vi "Simulation iRobot Sensors.vi"(8 "error in":errorcluster, 9 "Feedback Input":T1, 10 "Robot":T2, 11 "simulator":T16={"configuration"={"maxTime"=5.0, "enableVisualization"=TRUE, "Environment Definition"=path "simulation configuration.ini", "Record Location"=path "Simulation Record.xml", "autograde?"=TRUE, "interactive?"=FALSE, "Feedback Mode"=enum."debug navigation", "Robot State Charts"=[path "C:/Users/blueuser/Desktop/Robo Sim Berkley/cpsgrader-release-0.4/Simulators/EECS149lab/src/LabVIEW/statechart/Simulation Statechart.vi"], "statechart"=path "C:/Users/blueuser/Desktop/Robo Sim Berkley/cpsgrader-release-0.4/Simulators/EECS149lab/src/LabVIEW/statechart/Simulation Statechart.vi"}, "Statechart\ndisplay"=refnum, "first step?"=FALSE, "Robots Simulation Statecharts"=[], "Robots"=[]}) -> (0 "error out":errorcluster, 1 "Feedback Output":T1, 2 "sensors":T3={"net distance (mm)"=0, "net angle (deg)"=0, "accelerometer"={"x axis (g)"=0.0, "y axis (g)"=0.0, "z axis (g)"=0.0}, "iRobot Sensors"={"Bumps + Wheel Drops"={"Wheeldrop Caster"=FALSE, "Wheeldrop Left"=FALSE, "Wheeldrop Right"=FALSE, "Bump Left"=FALSE, "Bump Right"=FALSE}, "Wall"=FALSE, "Cliff Left"=FALSE, "Cliff Front Left"=FALSE, "Cliff Front Right"=FALSE, "Cliff Right"=FALSE, "Wall Signal"=0, "Cliff Left Signal"=0, "Cliff Front Left Signal"=0, "Cliff Front Right Signal"=0, "Cliff Right Signal"=0, "Buttons"={"Advance"=FALSE, "Play"=FALSE}, "Virtual Wall"=FALSE, "# Stream Packets"=0, "Requested Velocity (mm/s)"=0, "Requested Radius (mm)"=0, "Requested Right Wheel Velocity (mm/s)"=0, "Requested Left Wheel Velocity (mm/s)"=0, "Distance (mm)"=0, "Angle (deg)"=0, "Song Playing"=FALSE, "Song Number"=0, "Charging State"=enum."Not Charging", "Voltage (mV)"=0, "Current (mA)"=0, "Battery Temperature (deg C)"=0, "Battery Charge (mAh)"=0, "Battery Capacity (mAh)"=0, "Charging Sources"={"Internal Charger"=FALSE, "Home Base"=FALSE}, "OI Mode"=enum."Off", "Digital Inputs"={"Digital Input 0"=FALSE, "Digital Input 1"=FALSE, "Digital Input 2"=FALSE, "Digital Input 3"=FALSE, "Device Detect"=FALSE}, "Drivers & Wheel Overcurrent"={"Low-Side Driver 0"=FALSE, "Low-Side Driver 1"=FALSE, "Low-Side Driver 2"=FALSE, "Left Wheel"=FALSE, "Right Wheel"=FALSE}, "Analog Signal"=0, "Infrared"=255}, "Is Simulator?"=FALSE, "Kobuki Sensors"={"Bumps + Wheel Drops"={"Wheeldrop Left"=FALSE, "Wheeldrop Right"=FALSE, "Bump Left"=FALSE, "Bump Center"=FALSE, "Bump Right"=FALSE}, "Cliff Left"=FALSE, "Cliff Center"=FALSE, "Cliff Right"=FALSE, "Cliff Left Signal"=0, "Cliff Center Signal"=0, "Cliff Right Signal"=0, "Buttons"={"B0"=FALSE, "B1"=FALSE, "B2"=FALSE}, "# Stream Packets"=0, "Requested Velocity (mm/s)"=0, "Requested Radius (mm)"=0, "Requested Right Wheel Velocity (mm/s)"=0, "Requested Left Wheel Velocity (mm/s)"=0, "Left Wheel Encoder (ticks)"=0, "Angle (deg)"=0, "Song Playing"=FALSE, "Song Number"=0, "Charging State"=enum."Not Charging", "Voltage (mV)"=0, "Current (mA)"=0, "Battery Temperature (deg C)"=0, "Battery Charge (mAh)"=0, "Battery Capacity (mAh)"=0, "Charging Sources"={"Internal Charger"=FALSE, "Home Base"=FALSE}, "OI Mode"=enum."Off", "Digital Inputs"={"Digital Input 0"=FALSE, "Digital Input 1"=FALSE, "Digital Input 2"=FALSE, "Digital Input 3"=FALSE, "Device Detect"=FALSE}, "Drivers & Wheel Overcurrent"={"Low-Side Driver 0"=FALSE, "Low-Side Driver 1"=FALSE, "Low-Side Driver 2"=FALSE, "Left Wheel"=FALSE, "Right Wheel"=FALSE}, "Analog Signal"=0, "Infrared"=255, "Right Wheel Encoder (ticks) "=0, "TimeStamp"=0}} {"Kobuki Sensors"."Infrared" format="%02x"; "iRobot Sensors"."Infrared" format="%02x"; "accelerometer"."z axis (g)" format="%.3f"; "accelerometer"."y axis (g)" format="%.3f"; "accelerometer"."x axis (g)" format="%.3f"}, 3 "simulator":T16={"configuration"={"maxTime"=5.0, "enableVisualization"=TRUE, "Environment Definition"=path "simulation configuration.ini", "Record Location"=path "Simulation Record.xml", "autograde?"=TRUE, "interactive?"=FALSE, "Feedback Mode"=enum."debug navigation", "Robot State Charts"=[path "C:/Users/blueuser/Desktop/Robo Sim Berkley/cpsgrader-release-0.4/Simulators/EECS149lab/src/LabVIEW/statechart/Simulation Statechart.vi"], "statechart"=path "C:/Users/blueuser/Desktop/Robo Sim Berkley/cpsgrader-release-0.4/Simulators/EECS149lab/src/LabVIEW/statechart/Simulation Statechart.vi"}, "Statechart\ndisplay"=refnum, "first step?"=FALSE, "Robots Simulation Statecharts"=[], "Robots"=[]})   [LabVIEW 2014]
doc: "Simulates iRobot sensors. Automatically accumulates distance and angle."
uses:
  Simulator.ctl
  CyberSim interface/Simulation Configuration.ctl
  autograder/feedbackMode.ctl
  Multi Bot Code/RobotData.ctl
  <instrlib>/DC Motor Controller/HAIOL/DC Motor Controller.lvclass
  shared/Sensors.ctl
  iRobot/Sensor/Accelerometer.ctl
  iRobot/Sensor/Sensor Group 6.ctl
  iRobot/Sensor/Bumps + Wheel Drops.ctl
  iRobot/Sensor/Buttons.ctl
  iRobot/Sensor/Charging State.ctl
  iRobot/Sensor/Charging Sources Available.ctl
  iRobot/Sensor/OI Mode.ctl
  iRobot/Sensor/Cargo Bay Digital Inputs.ctl
  iRobot/Sensor/Low-Side Driver + Wheel Overcurrent.ctl
  Kobuki/KobukiSensors.ctl
  Kobuki/Kobuki Bumps and WheelDrops.ctl
  Kobuki/Kobuki Buttons.ctl
  Multi Bot Code/Sim Sensors Feedback.ctl
  <vilib>/Analysis/coordinate.llb/Angle Units.ctl
  <vilib>/Analysis/coordinate.llb/2D Cartesian Coordinate Rotation (Scalar).vi
  <vilib>/Analysis/coordinate.llb/Wrap Angle (scalar).vi
  <vilib>/Analysis/BLAS.llb/dnrm2 - Vector 2-Norm (DBL).vi
  <resource>/objmgr/LVODE.rc
  <vilib>/Analysis/NI_AALBLAS.lvlib
  <vilib>/robotics/Kinematics/NI_Kinematics.lvlib
  <vilib>/Analysis/NI_AAL_Angle.lvlib
  <vilib>/Analysis/NI_AALPro.lvlib
panel:
  # "Electrical: charging, battery, OI mode"
  # "Sensors: bump, cliff, button, wheel drop, wall, virtual wall"
  # "Motion: distance, angle, requested velocity"
  # "Cargo Bay: I/O, overcurrent, infrared"
  # "Song"
  # "Electrical: charging, battery, OI mode"
  # "Sensors: bump, cliff, button, wheel drop, wall, virtual wall"
  # "Motion: distance, angle, requested velocity"
  # "Cargo Bay: I/O, overcurrent, infrared"
  # "Song"
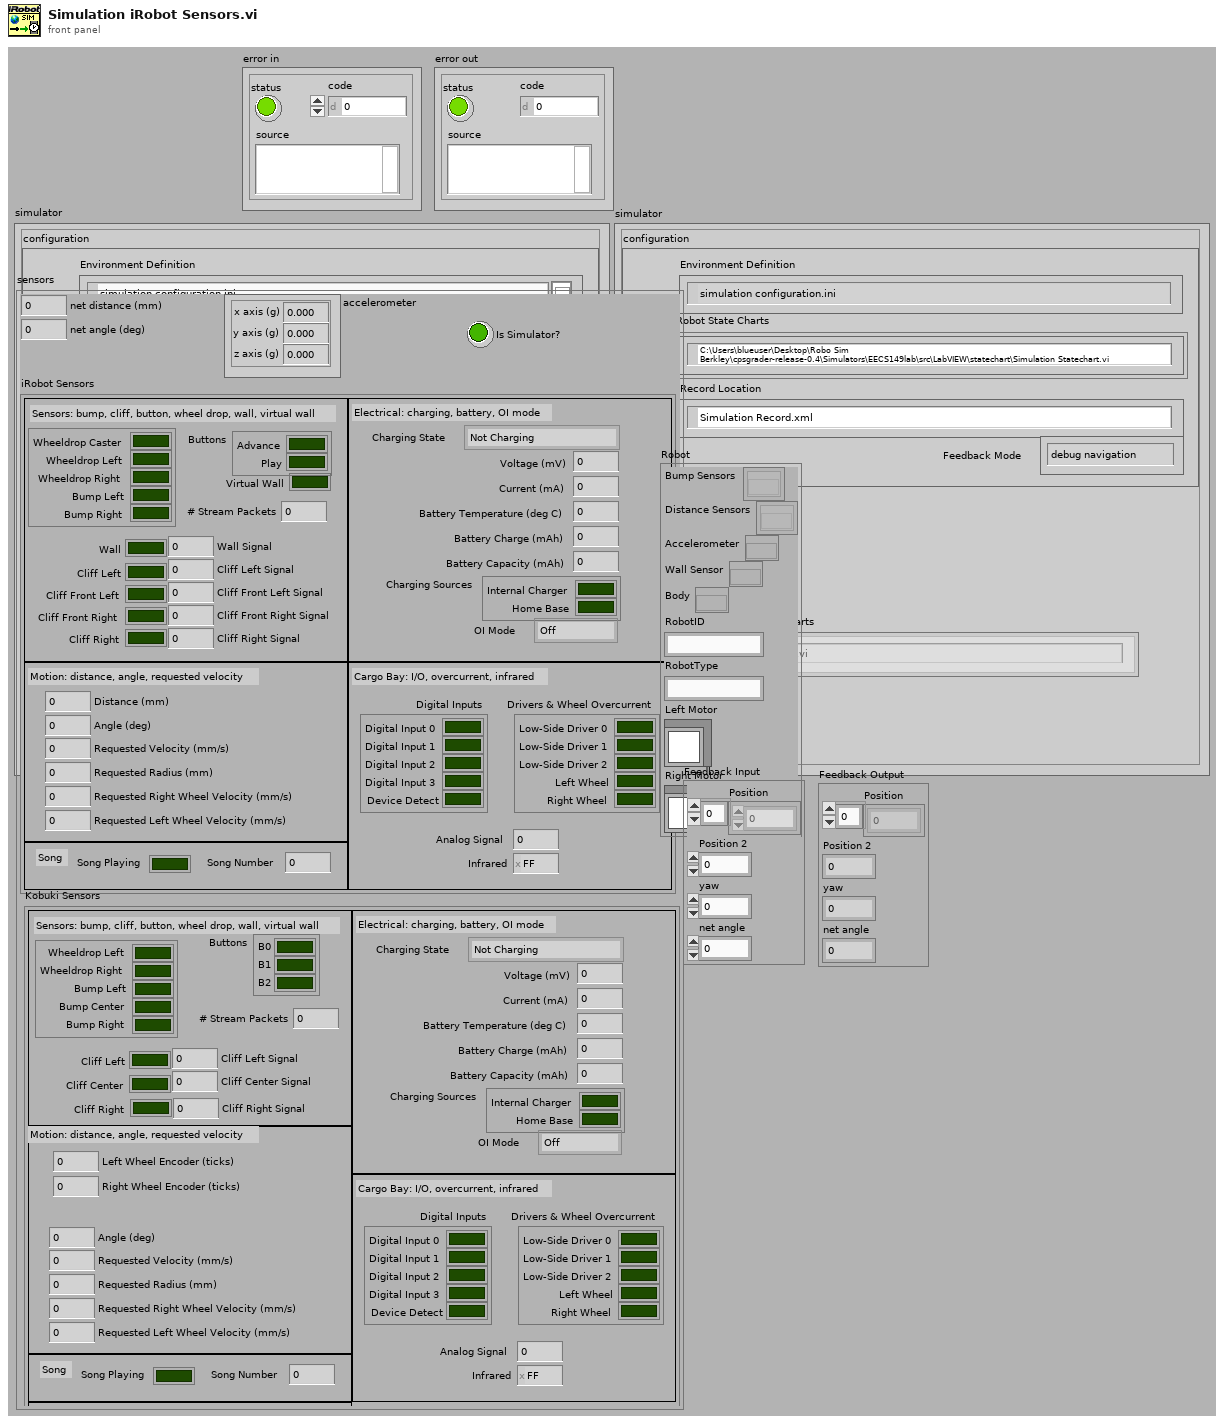
[diagram p1: front panel]
types:
  T1 = typedef "Sim Sensors Feedback.ctl" = cluster{"Position":sgl[], "Position 2":dbl, "yaw":dbl, "net angle":dbl}
  T2 = typedef "RobotData.ctl" = cluster{"Bump Sensors":refnum<k20>[], "Distance Sensors":refnum<k20>[], "Accelerometer":refnum<k20>, "Wall Sensor":refnum<k20>, "Body":refnum<k20>, "RobotID":string, "RobotType":string, "Left Motor":refnum<class "DC Motor Controller.lvclass">, "Right Motor":refnum<class "DC Motor Controller.lvclass">}
  T3 = typedef "Sensors.ctl" = cluster{"net distance (mm)":i32, "net angle (deg)":i32, "accelerometer":T4, "iRobot Sensors":T5, "Is Simulator?":bool, "Kobuki Sensors":T13}
  T4 = typedef "Accelerometer.ctl" = cluster{"x axis (g)":dbl, "y axis (g)":dbl, "z axis (g)":dbl}
  T5 = typedef "Sensor Group 6.ctl" = cluster{"Bumps + Wheel Drops":T6, "Wall":bool, "Cliff Left":bool, "Cliff Front Left":bool, "Cliff Front Right":bool, "Cliff Right":bool, "Wall Signal":u16, "Cliff Left Signal":u16, "Cliff Front Left Signal":u16, "Cliff Front Right Signal":u16, "Cliff Right Signal":u16, "Buttons":T7, "Virtual Wall":bool, "# Stream Packets":u8, "Requested Velocity (mm/s)":i16, "Requested Radius (mm)":i16, "Requested Right Wheel Velocity (mm/s)":i16, "Requested Left Wheel Velocity (mm/s)":i16, "Distance (mm)":i32, "Angle (deg)":i32, "Song Playing":bool, "Song Number":u8, "Charging State":T8, "Voltage (mV)":u16, "Current (mA)":i16, "Battery Temperature (deg C)":i8, "Battery Charge (mAh)":u16, "Battery Capacity (mAh)":u16, "Charging Sources":T9, "OI Mode":T10, "Digital Inputs":T11, "Drivers & Wheel Overcurrent":T12, "Analog Signal":u16, "Infrared":u8}
  T6 = typedef "Bumps + Wheel Drops.ctl" = cluster{"Wheeldrop Caster":bool, "Wheeldrop Left":bool, "Wheeldrop Right":bool, "Bump Left":bool, "Bump Right":bool}
  T7 = typedef "Buttons.ctl" = cluster{"Advance":bool, "Play":bool}
  T8 = typedef "Charging State.ctl" = enum16{"Not Charging", "Reconditioning Charging", "Full Charging", "Trickle Charging", "Waiting", "Charging Fault Condition"}
  T9 = typedef "Charging Sources Available.ctl" = cluster{"Internal Charger":bool, "Home Base":bool}
  T10 = typedef "OI Mode.ctl" = enum16{"Off", "Passive", "Safe", "Full"}
  T11 = typedef "Cargo Bay Digital Inputs.ctl" = cluster{"Digital Input 0":bool, "Digital Input 1":bool, "Digital Input 2":bool, "Digital Input 3":bool, "Device Detect":bool}
  T12 = typedef "Low-Side Driver + Wheel Overcurrent.ctl" = cluster{"Low-Side Driver 0":bool, "Low-Side Driver 1":bool, "Low-Side Driver 2":bool, "Left Wheel":bool, "Right Wheel":bool}
  T13 = typedef "KobukiSensors.ctl" = cluster{"Bumps + Wheel Drops":T14, "Cliff Left":bool, "Cliff Center":bool, "Cliff Right":bool, "Cliff Left Signal":u16, "Cliff Center Signal":u16, "Cliff Right Signal":u16, "Buttons":T15, "# Stream Packets":u8, "Requested Velocity (mm/s)":i16, "Requested Radius (mm)":i16, "Requested Right Wheel Velocity (mm/s)":i16, "Requested Left Wheel Velocity (mm/s)":i16, "Left Wheel Encoder (ticks)":i16, "Angle (deg)":i32, "Song Playing":bool, "Song Number":u8, "Charging State":T8, "Voltage (mV)":u16, "Current (mA)":i16, "Battery Temperature (deg C)":i8, "Battery Charge (mAh)":u16, "Battery Capacity (mAh)":u16, "Charging Sources":T9, "OI Mode":T10, "Digital Inputs":T11, "Drivers & Wheel Overcurrent":T12, "Analog Signal":u16, "Infrared":u8, "Right Wheel Encoder (ticks) ":i16, "TimeStamp":u16}
  T14 = typedef "Kobuki Bumps and WheelDrops.ctl" = cluster{"Wheeldrop Left":bool, "Wheeldrop Right":bool, "Bump Left":bool, "Bump Center":bool, "Bump Right":bool}
  T15 = typedef "Kobuki Buttons.ctl" = cluster{"B0":bool, "B1":bool, "B2":bool}
  T16 = typedef "Simulator.ctl" = cluster{"configuration":T17, "Statechart\ndisplay":refnum<vi>, "first step?":bool, "Robots Simulation Statecharts":path[], "Robots":T2[]}
  T17 = typedef "Simulation Configuration.ctl" = cluster{"maxTime":sgl, "enableVisualization":bool, "Environment Definition":path, "Record Location":path, "autograde?":bool, "interactive?":bool, "Feedback Mode":T18, "Robot State Charts":path[], "statechart":path}
  T18 = typedef "feedbackMode.ctl" = enum32{"debug navigation", "debug hill climb", "autograde navigation", "autograde hill climb"}
  T19 = typedef "NI_AAL_Angle.lvlib/Angle Units.ctl" = i32
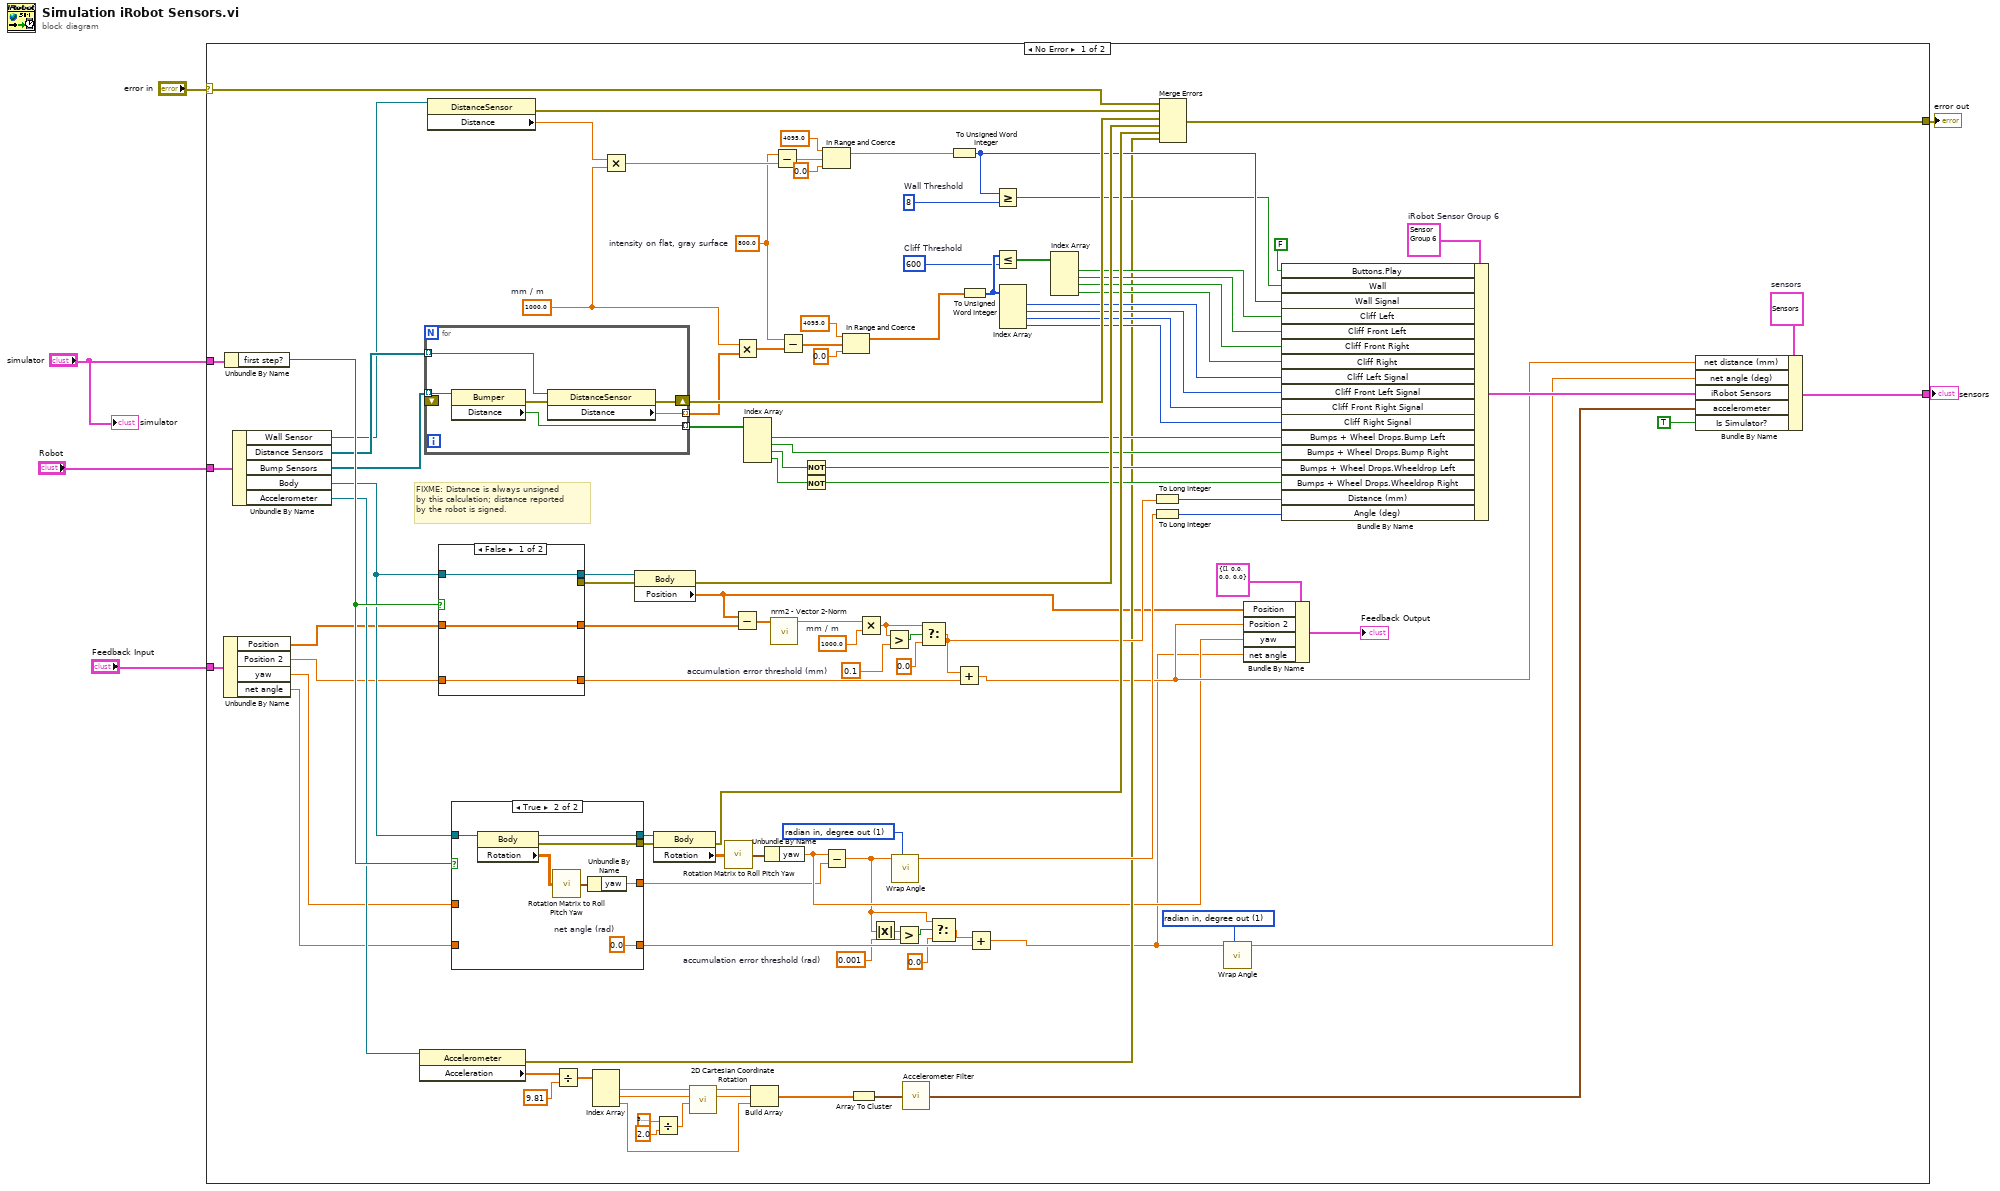
[diagram p0: block diagram]
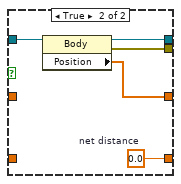
[diagram p2: hidden frame]
diagram:
  n1 = case shown="No Error" "error in" {
    selector: "error in" -> [w52 w142]
    tunnel: [w57 _] -> w6
    tunnel: "simulator" -> [w48 _]
    tunnel: [w53 w142] -> w5
    tunnel: "Robot" -> [w47 _]
    tunnel: "Feedback Input" -> [w35 _]
    frame No Error {
      w8 = 0.1  # accumulation error threshold (mm)
      w13 = 1000.0  # mm / m
      w18 = T19 1 items=["radian in, radian out", "radian in, degree out", "degree in, degree out", "degree in, radian out"] ("angle units")
      w21 = 0.001  # accumulation error threshold (rad)
      w58 = T3 {"net distance (mm)"=0, "net angle (deg)"=0, "accelerometer"={"x axis (g)"=0.0, "y axis (g)"=0.0, "z axis (g)"=0.0}, "iRobot Sensors"={"Bumps + Wheel Drops"={"Wheeldrop Caster"=FALSE, "Wheeldrop Left"=FALSE, "Wheeldrop Right"=FALSE, "Bump Left"=FALSE, "Bump Right"=FALSE}, "Wall"=FALSE, "Cliff Left"=FALSE, "Cliff Front Left"=FALSE, "Cliff Front Right"=FALSE, "Cliff Right"=FALSE, "Wall Signal"=0, "Cliff Left Signal"=0, "Cliff Front Left Signal"=0, "Cliff Front Right Signal"=0, "Cliff Right Signal"=0, "Buttons"={"Advance"=FALSE, "Play"=FALSE}, "Virtual Wall"=FALSE, "# Stream Packets"=0, "Requested Velocity (mm/s)"=0, "Requested Radius (mm)"=0, "Requested Right Wheel Velocity (mm/s)"=0, "Requested Left Wheel Velocity (mm/s)"=0, "Distance (mm)"=0, "Angle (deg)"=0, "Song Playing"=FALSE, "Song Number"=0, "Charging State"=enum."Not Charging", "Voltage (mV)"=0, "Current (mA)"=0, "Battery Temperature (deg C)"=0, "Battery Charge (mAh)"=0, "Battery Capacity (mAh)"=0, "Charging Sources"={"Internal Charger"=FALSE, "Home Base"=FALSE}, "OI Mode"=enum."Off", "Digital Inputs"={"Digital Input 0"=FALSE, "Digital Input 1"=FALSE, "Digital Input 2"=FALSE, "Digital Input 3"=FALSE, "Device Detect"=FALSE}, "Drivers & Wheel Overcurrent"={"Low-Side Driver 0"=FALSE, "Low-Side Driver 1"=FALSE, "Low-Side Driver 2"=FALSE, "Left Wheel"=FALSE, "Right Wheel"=FALSE}, "Analog Signal"=0, "Infrared"=0}, "Is Simulator?"=FALSE, "Kobuki Sensors"={"Bumps + Wheel Drops"={"Wheeldrop Left"=FALSE, "Wheeldrop Right"=FALSE, "Bump Left"=FALSE, "Bump Center"=FALSE, "Bump Right"=FALSE}, "Cliff Left"=FALSE, "Cliff Center"=FALSE, "Cliff Right"=FALSE, "Cliff Left Signal"=0, "Cliff Center Signal"=0, "Cliff Right Signal"=0, "Buttons"={"B0"=FALSE, "B1"=FALSE, "B2"=FALSE}, "# Stream Packets"=0, "Requested Velocity (mm/s)"=0, "Requested Radius (mm)"=0, "Requested Right Wheel Velocity (mm/s)"=0, "Requested Left Wheel Velocity (mm/s)"=0, "Left Wheel Encoder (ticks)"=0, "Angle (deg)"=0, "Song Playing"=FALSE, "Song Number"=0, "Charging State"=enum."Not Charging", "Voltage (mV)"=0, "Current (mA)"=0, "Battery Temperature (deg C)"=0, "Battery Charge (mAh)"=0, "Battery Capacity (mAh)"=0, "Charging Sources"={"Internal Charger"=FALSE, "Home Base"=FALSE}, "OI Mode"=enum."Off", "Digital Inputs"={"Digital Input 0"=FALSE, "Digital Input 1"=FALSE, "Digital Input 2"=FALSE, "Digital Input 3"=FALSE, "Device Detect"=FALSE}, "Drivers & Wheel Overcurrent"={"Low-Side Driver 0"=FALSE, "Low-Side Driver 1"=FALSE, "Low-Side Driver 2"=FALSE, "Left Wheel"=FALSE, "Right Wheel"=FALSE}, "Analog Signal"=0, "Infrared"=255, "Right Wheel Encoder (ticks) "=0, "TimeStamp"=0}}  # sensors
      w81 = u16 8  # Wall Threshold
      w82 = 800.0  # intensity on flat, gray surface
      w85 = T19 1 items=["radian in, radian out", "radian in, degree out", "degree in, degree out", "degree in, radian out"] ("angle units")
      w88 = 600  # Cliff Threshold
      w108 = T5 {"Bumps + Wheel Drops"={"Wheeldrop Caster"=FALSE, "Wheeldrop Left"=FALSE, "Wheeldrop Right"=FALSE, "Bump Left"=FALSE, "Bump Right"=FALSE}, "Wall"=FALSE, "Cliff Left"=FALSE, "Cliff Front Left"=FALSE, "Cliff Front Right"=FALSE, "Cliff Right"=FALSE, "Wall Signal"=0, "Cliff Left Signal"=0, "Cliff Front Left Signal"=0, "Cliff Front Right Signal"=0, "Cliff Right Signal"=0, "Buttons"={"Advance"=FALSE, "Play"=FALSE}, "Virtual Wall"=FALSE, "# Stream Packets"=0, "Requested Velocity (mm/s)"=0, "Requested Radius (mm)"=0, "Requested Right Wheel Velocity (mm/s)"=0, "Requested Left Wheel Velocity (mm/s)"=0, "Distance (mm)"=0, "Angle (deg)"=0, "Song Playing"=FALSE, "Song Number"=0, "Charging State"=enum."Not Charging", "Voltage (mV)"=0, "Current (mA)"=0, "Battery Temperature (deg C)"=0, "Battery Charge (mAh)"=0, "Battery Capacity (mAh)"=0, "Charging Sources"={"Internal Charger"=FALSE, "Home Base"=FALSE}, "OI Mode"=enum."Off", "Digital Inputs"={"Digital Input 0"=FALSE, "Digital Input 1"=FALSE, "Digital Input 2"=FALSE, "Digital Input 3"=FALSE, "Device Detect"=FALSE}, "Drivers & Wheel Overcurrent"={"Low-Side Driver 0"=FALSE, "Low-Side Driver 1"=FALSE, "Low-Side Driver 2"=FALSE, "Left Wheel"=FALSE, "Right Wheel"=FALSE}, "Analog Signal"=0, "Infrared"=0}  # iRobot Sensor Group 6
      w113 = 1000.0  # mm / m
      # "FIXME: Distance is always unsigned\nby this calculation; distance reported\nby the robot is signed."
      n2 = Unbundle By Name(w35) -> ("Position"=w34:sgl[], "Position 2"=w33:dbl, "yaw"=w32:dbl, "net angle"=w31:dbl)
      n3 = Unbundle By Name(w48) -> ("first step?"=w50:bool)
      n4 = Unbundle By Name(w47) -> ("Wall Sensor"=w42:refnum<k20>, "Distance Sensors"=w43:refnum<k20>[], "Bump Sensors"=w44:refnum<k20>[], "Body"=w45:refnum<k20>, "Accelerometer"=w46:refnum<k20>)
      n5 = property class="Accelerometer"(reference=w46) -> (error out=w51:errorcluster, "Acceleration"=w72:sgl[])  [unwired: 1 in, 1 out]
      n6 = for {
        tunnel: [w141] -> w103 mode=indexing
        tunnel: w44 -> [w140] mode=indexing
        tunnel: [w139] -> w114 mode=indexing
        shift-right: [w137] -> w111
        shift-left: _ -> [_]
        tunnel: w43 -> [w136] mode=indexing
        n7 = property class="Bumper"(reference=w140) -> (error out=w138:errorcluster, "Distance"=w139:bool)  [unwired: 1 in, 1 out]
        n8 = property class="DistanceSensor"(reference=w136, error in=w138) -> (error out=w137:errorcluster, "Distance"=w141:sgl)  [unwired: 1 out]
      }
      n9 = property class="DistanceSensor"(reference=w42) -> (error out=w112:errorcluster, "Distance"=w117:sgl)  [unwired: 1 in, 1 out]
      n10 = case shown="False" w50 {
        tunnel: w45 -> [w119 w125]
        tunnel: [w120 w122] -> w15
        tunnel: w34 -> [w120 _]
        tunnel: [_ w124] -> w16
        tunnel: [w119 w123] -> w17
        tunnel: w33 -> [w118 _]
        tunnel: [w118 w121] -> w11
        frame False {
        }
        frame True {
          w121 = 0.0  # net distance
          n11 = property class="Body"(reference=w125) -> (reference out=w123:refnum<k20>, error out=w124:errorcluster, "Position"=w122:sgl[])  [unwired: 1 in]
        }
      }
      n12 = case shown="True" w50 {
        tunnel: w45 -> [w128 w135]
        tunnel: [w128 w134] -> w30
        tunnel: [_ w133] -> w29
        tunnel: [w127 w130] -> w26
        tunnel: w32 -> [w127 _]
        tunnel: [w126 w129] -> w23
        tunnel: w31 -> [w126 _]
        frame False {
        }
        frame True {
          w129 = 0.0  # net angle (rad)
          n13 = property class="Body"(reference=w135) -> (reference out=w134:refnum<k20>, error out=w133:errorcluster, "Rotation"=w132:sgl[][])  [unwired: 1 in]
          n14 = call <vilib>:"Rotation Matrix to Roll Pitch Yaw.vi"("rotation matrix"=w132) -> ("angles"=w131:cluster{"roll":dbl, "pitch":dbl, "yaw":dbl})
          n15 = Unbundle By Name(w131) -> ("yaw"=w130:dbl)
        }
      }
      n16 = Divide(x=w72, y=9.81) -> (x/y=w70:dbl[])
      n17 = Index Array(array=w70) -> (element #1=w69:dbl, element #2=w68:dbl, element #3=w62:dbl)  [unwired: 3 in]
      n18 = Multiply(x=w117, y=w113) -> (x*y=w83:dbl)
      n19 = property class="Body"(reference=w17, error in=w16) -> (error out=w110:errorcluster, "Position"=w41:sgl[])  [unwired: 1 out]
      n20 = property class="Body"(reference=w30, error in=w29) -> (error out=w109:errorcluster, "Rotation"=w28:sgl[][])  [unwired: 1 out]
      n21 = Divide(x=3.141592653589793, y=2.0) -> (x/y=w65:dbl)
      n22 = call-poly <vilib>:"2D Cartesian Coordinate Rotation.vi"("theta"=w65, "y"=w68, "x"=w69) -> ("y out"=w63:dbl, "x out"=w64:dbl)  [unwired: 6 in, 1 out]
      n23 = call <vilib>:"Rotation Matrix to Roll Pitch Yaw.vi"("rotation matrix"=w28) -> ("angles"=w27:cluster{"roll":dbl, "pitch":dbl, "yaw":dbl})
      n24 = Subtract(x=w41, y=w15) -> (x-y=w12:sgl[])
      n25 = Multiply(x=w113, y=w103) -> (x*y=w84:dbl[])
      n26 = Index Array(array=w114) -> (element #1=w107:bool, element #2=w106:bool, element #3=w116:bool, element #4=w115:bool)  [unwired: 4 in]
      n27 = Build Array(w64, w63, w62) -> (w61:dbl[])
      n28 = Unbundle By Name(w27) -> ("yaw"=w39:dbl)
      n29 = call-poly <vilib>:"nrm2 - Vector 2-Norm.vi"("x"=w12) -> ("dnrm2"=w14:dbl)  [unwired: 9 in, 1 out]
      n30 = Subtract(x=w82, y=w83) -> (x-y=w80:dbl)
      n31 = Subtract(x=w82, y=w84) -> (x-y=w74:dbl[])
      n32 = Not(x=w116) -> (.not. x?=w105:bool)
      n33 = Not(x=w115) -> (.not. x?=w104:bool)
      n34 = In Range and Coerce(upper limit=4095.0, x=w80, lower limit=0.0) -> (coerced(x)=w77:dbl)  [unwired: 1 out]
      n35 = Subtract(x=w39, y=w26) -> (x-y=w19:dbl)
      n36 = In Range and Coerce(upper limit=4095.0, x=w74, lower limit=0.0) -> (coerced(x)=w73:dbl[])  [unwired: 1 out]
      n37 = Array To Cluster(array=w61) -> (cluster=w55:cluster{"[0]":dbl, "[1]":dbl, "[2]":dbl})
      n38 = Multiply(x=w14, y=w13) -> (x*y=w10:dbl)
      n39 = Absolute Value(x=w19) -> (abs(x)=w20:dbl)
      n40 = Greater?(x=w10, y=w8) -> (0:w9:bool)
      n41 = call-poly <vilib>:"Wrap Angle.vi"("angle units"=w18, "angle in"=w19) -> ("angle out"=w95:dbl)  [unwired: 8 in, 1 out]
      n42 = Greater?(x=w20, y=w21) -> (0:w25:bool)
      n43 = call "Accelerometer Filter.vi"("accelerometer (g)"=w55) -> ("filtered accelerometer (g)"=w54:T4)  [unwired: 3 in]
      n44 = Select(t=w10, s=w9, f=0.0) -> (s? t:f=w97:dbl)
      n45 = Select(t=w19, s=w25, f=0.0) -> (s? t:f=w24:dbl)
      n46 = To Unsigned Word Integer(number=w77) -> (unsigned 16bit integer=w87:u16)
      n47 = Add(x=w97, y=w11) -> (x+y=w40:dbl)
      n48 = To Unsigned Word Integer(number=w73) -> (unsigned 16bit integer=w94:u16[])
      n49 = Add(x=w24, y=w23) -> (x+y=w38:dbl)
      n50 = Greater Or Equal?(x=w87, y=w81) -> (x >= y?=w86:bool)
      n51 = Less Or Equal?(x=w94, y=w88) -> (x <= y?=w93:bool[])
      n52 = Index Array(array=w94) -> (element #1=w102:u16, element #2=w101:u16, element #3=w100:u16, element #4=w99:u16)  [unwired: 4 in]
      n53 = Index Array(array=w93) -> (element #1=w89:bool, element #2=w90:bool, element #3=w91:bool, element #4=w92:bool)  [unwired: 4 in]
      n54 = To Long Integer(number=w97) -> (32bit integer=w98:i32)
      n55 = To Long Integer(number=w95) -> (32bit integer=w96:i32)
      n56 = Merge Errors(w52, w112, w111, w110, w109, w51) -> (w53:errorcluster)
      n57 = call-poly <vilib>:"Wrap Angle.vi"("angle units"=w85, "angle in"=w38) -> ("angle out"=w59:dbl)  [unwired: 8 in, 1 out]
      n58 = Bundle By Name(cluster=T1 {"Position"=[], "Position 2"=0.0, "yaw"=0.0, "net angle"=0.0} ("output cluster"), "Position"=w41, "Position 2"=w40, "yaw"=w39, "net angle"=w38) -> (→"Feedback Output":T1)
      n59 = Bundle By Name(cluster=w108, "Buttons.Play"=FALSE, "Wall"=w86, "Wall Signal"=w87, "Cliff Left"=w89, "Cliff Front Left"=w90, "Cliff Front Right"=w91, "Cliff Right"=w92, "Cliff Left Signal"=w102, "Cliff Front Left Signal"=w101, "Cliff Front Right Signal"=w100, "Cliff Right Signal"=w99, "Bumps + Wheel Drops.Bump Left"=w107, "Bumps + Wheel Drops.Bump Right"=w106, "Bumps + Wheel Drops.Wheeldrop Left"=w105, "Bumps + Wheel Drops.Wheeldrop Right"=w104, "Distance (mm)"=w98, "Angle (deg)"=w96) -> (w60:T5)
      n60 = Bundle By Name(cluster=w58, "net distance (mm)"=w40, "net angle (deg)"=w59, "iRobot Sensors"=w60, "accelerometer"=w54, "Is Simulator?"=TRUE) -> (w57:T3)
    }
    frame Error {
    }
  }
  "error out" <- w5
  "sensors" <- w6
  "simulator" <- "simulator"
